vi "strac H.vi"() -> ()   [LabVIEW 2020]
panel:
  out "Numeric 6":i32
  out "Numeric 5":i32
  out "Numeric 4":i32
  out "Array 13":dbl[](array[numeric])
  out "Array 12":dbl[](array[numeric])
  out "Numeric 3":i32
  out "Array 11":string[](array[string])
  out "String":string
  out "Array 10":i32[](array[numeric])
  out "Numeric 2":dbl
  in  "Array 8":dbl[](array[numeric])
  out "Array 7":i32[](array[numeric])
  out "Array 6":dbl[](array[numeric])
  in  "Array 5":dbl[](array[numeric])
  out "Array 4":i32[](array[numeric])
  out "Numeric":dbl
  out "Array 2":i32[](array[numeric])
  in  "Array":dbl[](array[numeric])
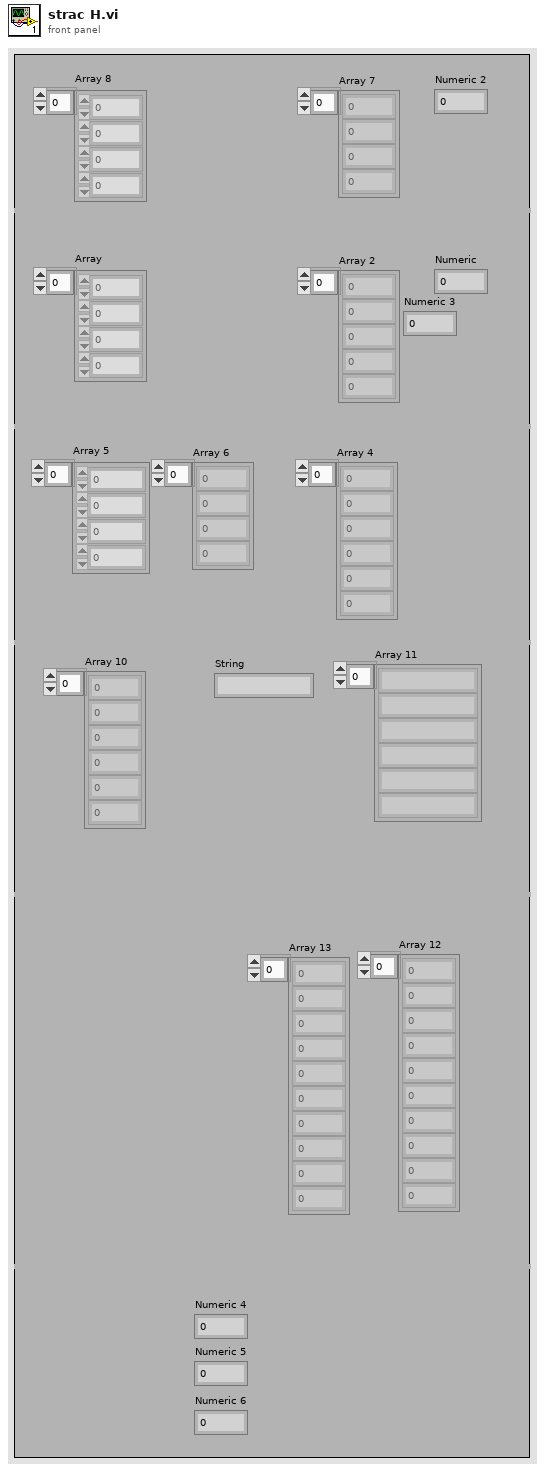
[diagram p1: front panel]
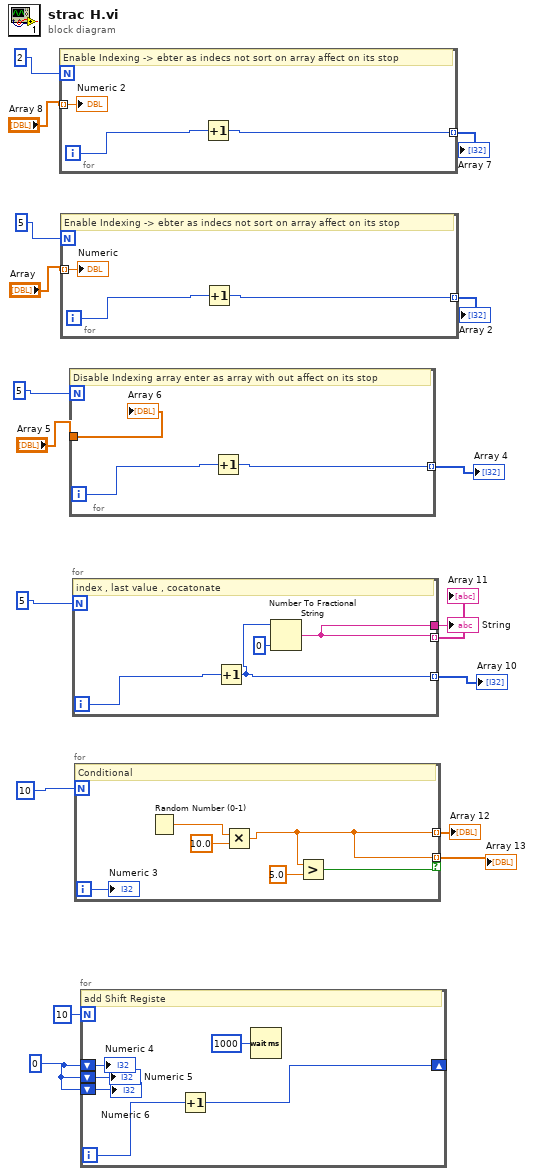
[diagram p0: block diagram]
diagram:
  w1 = 0
  n1 = for {
    N: 2 -> [_]
    tunnel: "Array 8" -> [w19] mode=indexing
    tunnel: [w20] -> w12 mode=indexing
    i -> [w21]
    # "Enable Indexing -> ebter as indecs not sort on array affect on its stop"
    n2 = Increment(x=w21) -> (x+1=w20:i32)
    "Numeric 2" <- w19
  }
  "Array 7" <- w12
  n3 = for {
    N: 5 -> [_]
    tunnel: "Array" -> [w22] mode=indexing
    tunnel: [w23] -> w16 mode=indexing
    i -> [w24]
    # "Enable Indexing -> ebter as indecs not sort on array affect on its stop"
    n4 = Increment(x=w24) -> (x+1=w23:i32)
    "Numeric" <- w22
  }
  "Array 2" <- w16
  n5 = for {
    N: 5 -> [_]
    tunnel: "Array 5" -> [w25]
    tunnel: [w26] -> w13 mode=indexing
    i -> [w27]
    # "Disable Indexing array enter as array with out affect on its stop"
    n6 = Increment(x=w27) -> (x+1=w26:i32)
    "Array 6" <- w25
  }
  "Array 4" <- w13
  n7 = for {
    N: 5 -> [_]
    tunnel: [w29] -> w9 mode=indexing
    tunnel: [w28] -> w7
    tunnel: [w28] -> w6 mode=indexing
    i -> [w31]
    # "index , last value , cocatonate"
    n8 = Increment(x=w31) -> (x+1=w29:i32)
    n9 = Number To Fractional String(number=w29, precision (6)=i16 0) -> (F-format string=w28:string)  [unwired: 2 in]
  }
  "Array 10" <- w9
  "String" <- w7
  "Array 11" <- w6
  n10 = for {
    N: 10 -> [_]
    tunnel: [w33] -> w4 mode=indexing
    tunnel: [w33] -> w3 mode=indexing if=w34
    i -> [w37]
    # "Conditional"
    n11 = Random Number (0-1)() -> (number: 0 to 1=w36:dbl)
    n12 = Multiply(x=w36, y=10.0) -> (x*y=w33:dbl)
    n13 = Greater?(x=w33, y=5.0) -> (0:w34:bool)
    "Numeric 3" <- w37
  }
  "Array 12" <- w4
  "Array 13" <- w3
  n14 = for {
    N: 10 -> [_]
    shift-right: [w42] -> _
    shift-left: w1 -> [w41]
    shift-left: w1 -> [w39]
    shift-left: w1 -> [w40]
    i -> [w43]
    # "add Shift Registe"
    n15 = Increment(x=w43) -> (x+1=w42:i32)
    n16 = Wait (ms)(milliseconds to wait=u32 1000) -> ()  [unwired: 1 out]
    "Numeric 4" <- w41
    "Numeric 5" <- w39
    "Numeric 6" <- w40
  }
